vi "VOL.vi"(0 "System no.":i32=1 min=1 max=4 step=1, 2 "PZT channel":string[](array[string]), 3 "PZT voltage":dbl[](array[numeric]) format="%.6f", 4 "No.of digits":i16=4, 5 "error in":errorcluster) -> (19 "error out":errorcluster)   [LabVIEW 2020]
doc: "Sets absolute PZT voltage for specified piezo channel. No. of digits is the number of digits after the decimal point in the voltage value(s) that will be sent. If the commanded voltage exceeds the voltage limits of the piezo channel, then the command is not executed.\n\nAnalog system: PZT channel is identical with axis ID.\nE-761: PZT channel can be 1 to 4."
panel:
  # "Sets absolute PZT voltage for specified piezo channel."
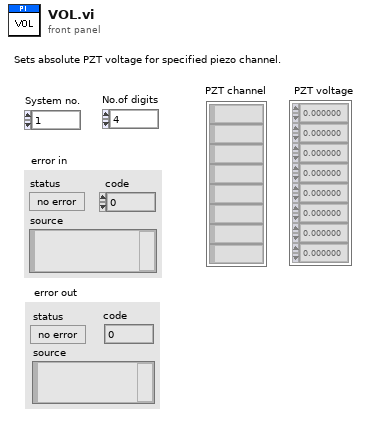
[diagram p1: front panel]
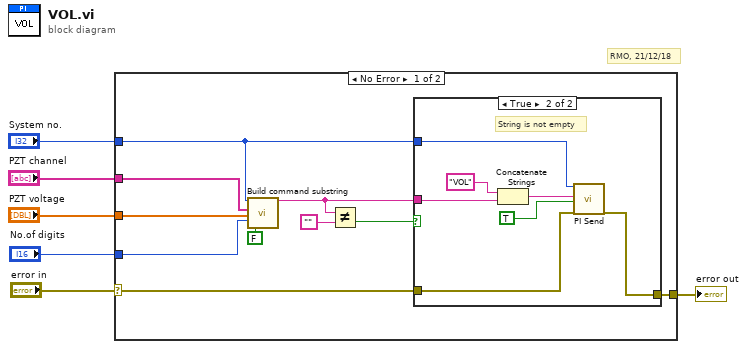
[diagram p0: block diagram]
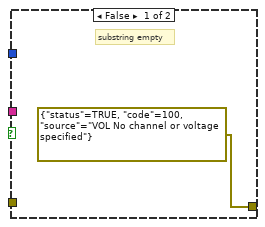
[diagram p2: hidden frame]
diagram:
  # "RMO, 21/12/18"
  n1 = case shown="No Error" "error in" {
    selector: "error in" -> [w7 w25]
    tunnel: [w16 w25] -> w6
    tunnel: "PZT voltage" -> [w13 _]
    tunnel: "No.of digits" -> [w12 _]
    tunnel: "System no." -> [w9 _]
    tunnel: "PZT channel" -> [w11 _]
    frame No Error {
      n2 = call "Build command substring.vi"("System no."=w9, "Affected axes"=w11, "Parameters"=w13, "No. of digits"=w12, "Parameter no. format \n(Decimal: FALSE)"=FALSE ("Parameter no. format \n(Decimal: FALSE)")) -> ("Command substring"=w14:string)  [unwired: 2 in, 12 out]
      n3 = Not Equal?(x=w14, y="") -> (x != y?=w10:bool)
      n4 = case shown="True" w10 {
        tunnel: w14 -> [_ w23]
        tunnel: [errorcluster {"status"=TRUE, "code"=100, "source"="VOL No channel or voltage specified"} ("error out") w19] -> w16
        tunnel: w7 -> [_ w20]
        tunnel: w9 -> [_ w18]
        frame False {
          # "substring empty"
        }
        frame True {
          # "String is not empty"
          n5 = Concatenate Strings("VOL", w23) -> (w21:string)
          n6 = call "PI Send.vi"("System no."=w18, "String to send"=w21, "Attach termination char.?"=TRUE ("Attach Linefeed?"), "error in"=w20) -> ("error out"=w19:errorcluster)  [unwired: 2 in, 13 out]
        }
      }
    }
    frame Error {
    }
  }
  "error out" <- w6
